vi "Get VI Common Properties.vi"(8 "错误输入（无错误）":errorcluster, 11 "VI Ref In":refnum<vi>) -> (0 "错误输出":errorcluster, 2 "VI Common Prop":T1, 3 "VI Ref Out":refnum<vi>)   [LabVIEW 2012, in "VIRef.lvlib"]
uses:
  VIRef.lvlib
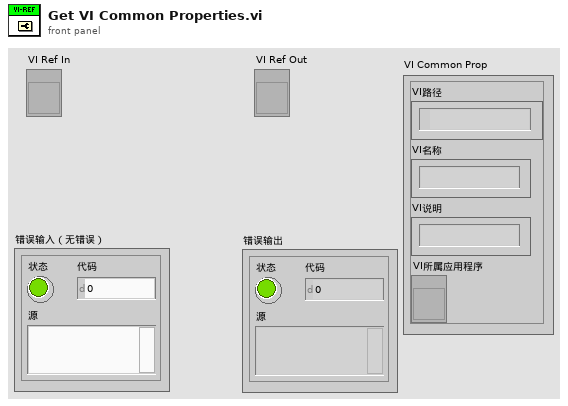
[diagram p1: front panel]
types:
  T1 = cluster{"VI路径":path, "VI名称":string, "VI说明":string, "VI所属应用程序":refnum<vi>}
  T2 = cluster{"Path":path, "Name":string, "Description":string, "OwningApp":refnum<vi>}
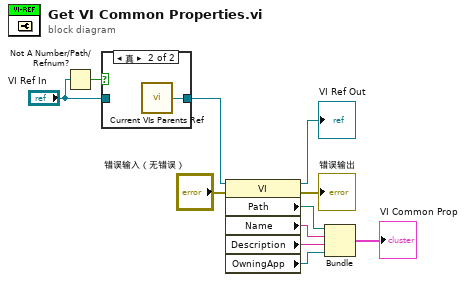
[diagram p0: block diagram]
diagram:
  n1 = Not A Number/Path/Refnum?(number/path/refnum="VI Ref In") -> (NaN/Path/Refnum?=w11:bool)
  n2 = case shown="真" w11 {
    tunnel: [w12 w13] -> w7
    tunnel: "VI Ref In" -> [w12 _]
    frame False {
    }
    frame True {
      n3 = call "Current VIs Parents Ref.vi"() -> ("Calling VI's Reference"=w13:refnum<vi>)  [unwired: 2 in]
    }
  }
  n4 = property class="VI"(reference=w7, error in="错误输入（无错误）") -> (reference out=→"VI Ref Out":refnum<vi>, error out=→"错误输出":errorcluster, "Path"=w5:path, "Name"=w4:string, "Description"=w3:string, "OwningApp"=w2:refnum<vi>)
  n5 = Bundle("Path"=w5, "Name"=w4, "Description"=w3, "OwningApp"=w2) -> (→"VI Common Prop":T2)  [unwired: 1 in]
